vi "Calculate Angle from Position.vi"(5 "Angle Array":dbl[](array[numeric])=[5.0, 7.0, 10.0, 12.0, 15.0, 17.0, 20.0, 22.0, 25.0, 27.0, 30.0, 37.0, 40.0], 7 "Position Array":i32[](array[numeric])=[100, 142, 184, 226, 268, 290, 332, 374, 416, 458, 500, 542, 584], 11 "Sensor Unit Position":i32) -> (3 "Current Angle":dbl)   [LabVIEW 2020, in "Angler_ACT.lvlib"]
uses:
  Angler_ACT.lvlib
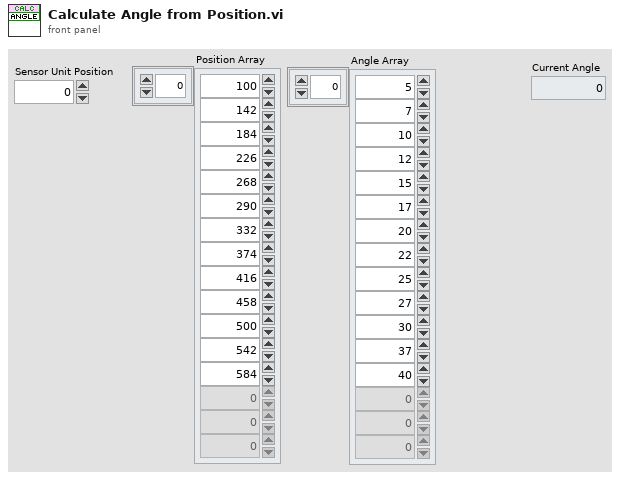
[diagram p1: front panel]
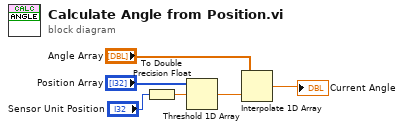
[diagram p0: block diagram]
diagram:
  n1 = To Double Precision Float(number="Sensor Unit Position") -> (double precision float=w1:dbl)
  n2 = Threshold 1D Array(2:w1, 3:"Position Array") -> (0:w4:dbl)  [unwired: 1 in]
  n3 = Interpolate 1D Array(1:w4, 2:"Angle Array") -> (0:→"Current Angle":dbl)
